vi "Add Object Parameter - Known Type.vi"(5 "JSON Compatible Type":T1=enum."Unknown", 6 "Add Parameter as JSON Tree?":bool, 7 "JSON Type":T2=enum."Unknown", 8 "error in (no error)":errorcluster, 9 "Name":string, 10 "Value":variant, 11 "JSON Tree in (JSON Object)":variant) -> (0 "error out":errorcluster, 3 "JSON Tree out (JSON Object)":variant)   [LabVIEW 2014, in "i3-json.lvlib"]
doc: "Adds a new value of a known type to the JSON Tree"
uses:
  i3-json.lvlib
  JSON Types/JSON Type.ctl
  JSON Types/JSON Compatible Type.ctl
  Error Handling/Throw JSON Error Files/Throw JSON Error - Invalid Type Error.vi
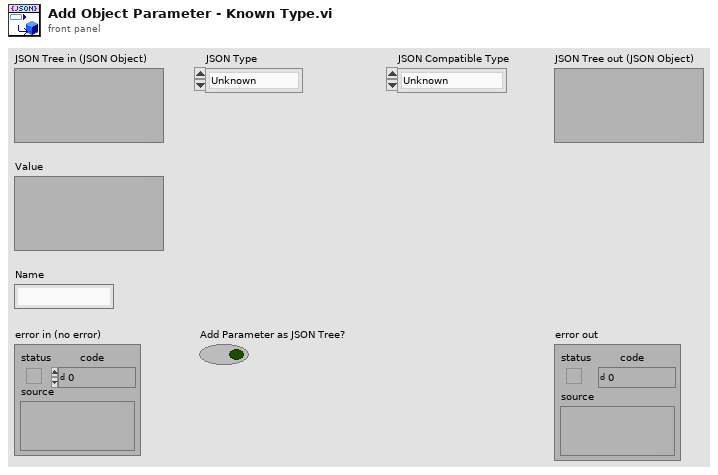
[diagram p1: front panel]
types:
  T1 = typedef "i3-json.lvlib/JSON Compatible Type.ctl" = enum16{"1D Double Array", "1D String Array", "1D Boolean Array", "Unknown"}
  T2 = typedef "i3-json.lvlib/JSON Type.ctl" = enum8{"JSON Compatible", "JSON Array", "JSON Object", "JSON Null", "Double", "String", "Boolean", "Unknown"}
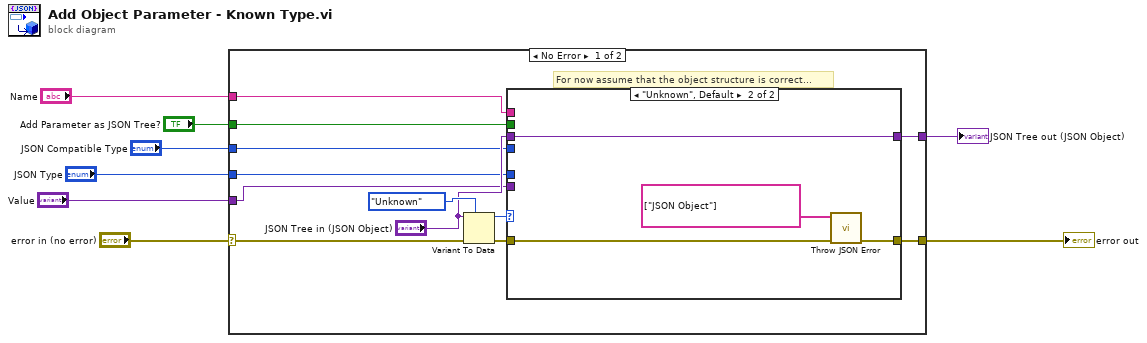
[diagram p0: block diagram]
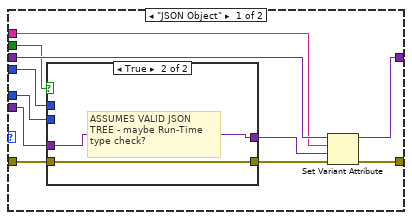
[diagram p2: hidden frame]
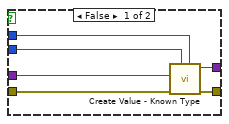
[diagram p3: hidden frame]
diagram:
  n1 = case shown="No Error" "error in (no error)" {
    selector: "error in (no error)" -> [w17 w44]
    tunnel: [w16 w44] -> w7
    tunnel: [w14 _] -> w6
    tunnel: "Name" -> [w13 _]
    tunnel: "Value" -> [w12 _]
    tunnel: "Add Parameter as JSON Tree?" -> [w11 _]
    tunnel: "JSON Compatible Type" -> [w10 _]
    tunnel: "JSON Type" -> [w9 _]
    frame No Error {
      # "For now assume that the object structure is correct..."
      n2 = Variant To Data(error in=w17, type=JSON_Type."Unknown" ("JSON Type"), Variant="JSON Tree in (JSON Object)") -> (data=w19:T2, error out=w15:errorcluster)
      n3 = case shown="\"Unknown\", Default" w19 {
        tunnel: "JSON Tree in (JSON Object)" -> [w26 w43]
        tunnel: w15 -> [w27 w41]
        tunnel: [w29 w43] -> w14
        tunnel: [w28 w40] -> w16
        tunnel: w13 -> [w25 _]
        tunnel: w12 -> [w24 _]
        tunnel: w11 -> [w23 _]
        tunnel: w10 -> [w22 _]
        tunnel: w9 -> [w21 _]
        frame "JSON Object" {
          n4 = case shown="True" w23 {
            tunnel: [w37 w38] -> w31
            tunnel: [w36 w39] -> w30
            tunnel: w27 -> [w35 w38]
            tunnel: w24 -> [w34 w39]
            tunnel: w22 -> [w33 _]
            tunnel: w21 -> [w32 _]
            frame False {
              n5 = call "Create Value - Known Type.vi"("JSON Compatible Type"=w33, "JSON Type"=w32, "error in (no error)"=w35, "Value"=w34) -> ("error out"=w37:errorcluster, "JSON Tree"=w36:variant)  [unwired: 6 in]
            }
            frame True {
              # "ASSUMES VALID JSON\nTREE - maybe Run-Time\ntype check?"
            }
          }
          n6 = Set Variant Attribute(Variant=w26, name=w25, value=w30, error in=w31) -> (Variant out=w29:variant, error out=w28:errorcluster)  [unwired: 1 out]
        }
        frame "Unknown", Default {
          n7 = call-poly "Throw JSON Error.vi"("error in (no error)"=w41, "Valid Types"=string[] ["JSON Object"]) -> ("error out"=w40:errorcluster)  [unwired: 9 in]
        }
      }
    }
    frame Error {
    }
  }
  "error out" <- w7
  "JSON Tree out (JSON Object)" <- w6
